vi "Abort Output Trigger.vi"(8 "error in (no error)":errorcluster {"code" format="%.0x"}, 10 "Channel Name (1)":string="1", 11 "VISA resource name":refnum<visa-resource-name>) -> (0 "error out":errorcluster {"code" format="%.0x"}, 3 "VISA resource name out":refnum<visa-resource-name>)   [LabVIEW 2018, in "Agilent N6700 Series.lvlib"]
doc: "Aborts all pending output changes if the power supply is currently waiting for a trigger to change the output signal.\n\nIf the power supply is not waiting for a trigger, this VI does nothing."
uses:
  Agilent N6700 Series.lvlib
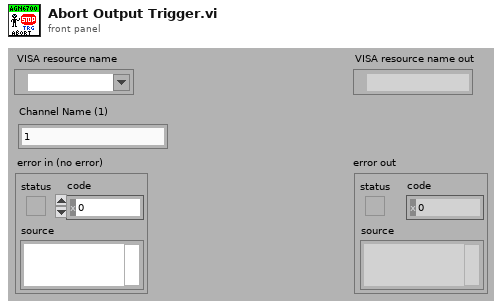
[diagram p1: front panel]
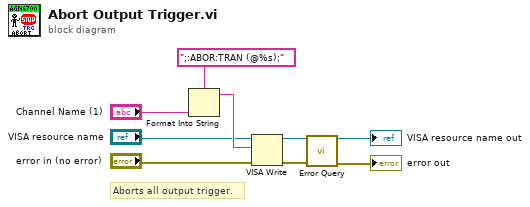
[diagram p0: block diagram]
diagram:
  # "Aborts all output trigger."
  n1 = Format Into String(format string=";:ABOR:TRAN (@%s);", "Channel Name (1)") -> (resulting string=w8:string)  [unwired: 2 in, 1 out]
  n2 = VISA Write(VISA resource name="VISA resource name", write buffer=w8, error in (no error)="error in (no error)") -> (VISA resource name out=w5:refnum<visa-resource-name>, error out=w4:errorcluster)  [unwired: 1 out]
  n3 = call "Error Query.vi"("VISA resource name"=w5, "error in (no error)"=w4) -> ("VISA resource name out"=→"VISA resource name out":refnum<visa-resource-name>, "error out"=→"error out":errorcluster)  [unwired: 10 in, 2 out]
